vi "Asynchronous Dialog Launcher.vi"(4 "Python Message ID":i32, 7 "Server Alias":string, 8 "error in (no error)":errorcluster, 10 "Data":string[](array[string]), 11 "Script ID":i64) -> (0 "error out":errorcluster)   [LabVIEW 2013]
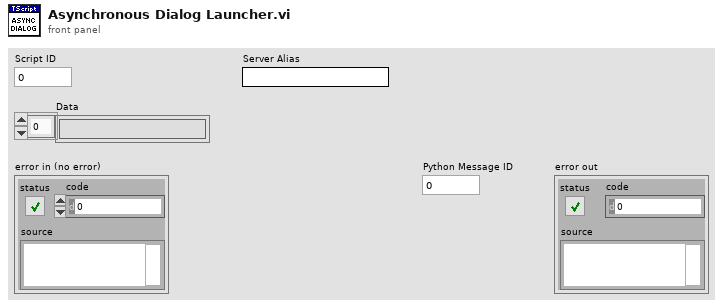
[diagram p1: front panel]
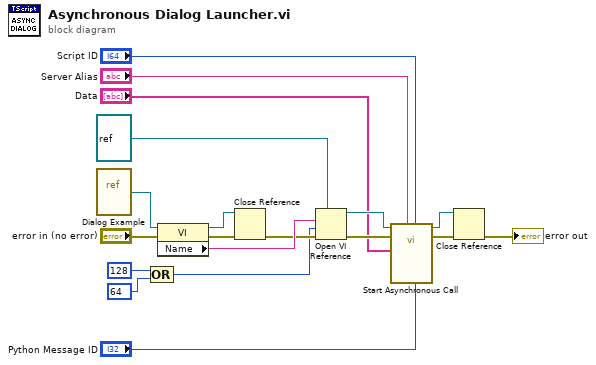
[diagram p0: block diagram]
diagram:
  n1 = vi-ref "Dialog Example.vi"() -> (w18:refnum<vi>)
  n2 = Compound Arithmetic op=OR(128 ("options"), 64 ("options")) -> (w1:i32)
  n3 = property class="VI"(reference=w18, error in="error in (no error)") -> (reference out=w7:refnum<vi>, error out=w8:errorcluster, "Name"=w19:string)
  n4 = Close Reference(reference=w7, error in (no error)=w8) -> (error out=w6:errorcluster)
  n5 = Open VI Reference(type specifier VI Refnum (for type only)=refnum<vi> refnum, vi path=w19, options=w1, error in (no error)=w6) -> (vi reference=w14:refnum<vi>, error out=w16:errorcluster)  [unwired: 2 in]
  n6 = call-by-ref "Start Asynchronous Call"(reference=w14, error in=w16, "Python Message ID"="Python Message ID", "Script ID"="Script ID", "Server Alias"="Server Alias", "Choices"="Data") -> (reference out=w10:refnum<vi>, error out=w11:errorcluster)  [unwired: 6 in, 2 out]
  n7 = Close Reference(reference=w10, error in (no error)=w11) -> (error out=→"error out":errorcluster)
